vi "Base File Path.vi"() -> (3 "Paths Out":T1)   [LabVIEW 2018]
uses:
  File Paths.ctl
panel:
  in  "Paths":T1
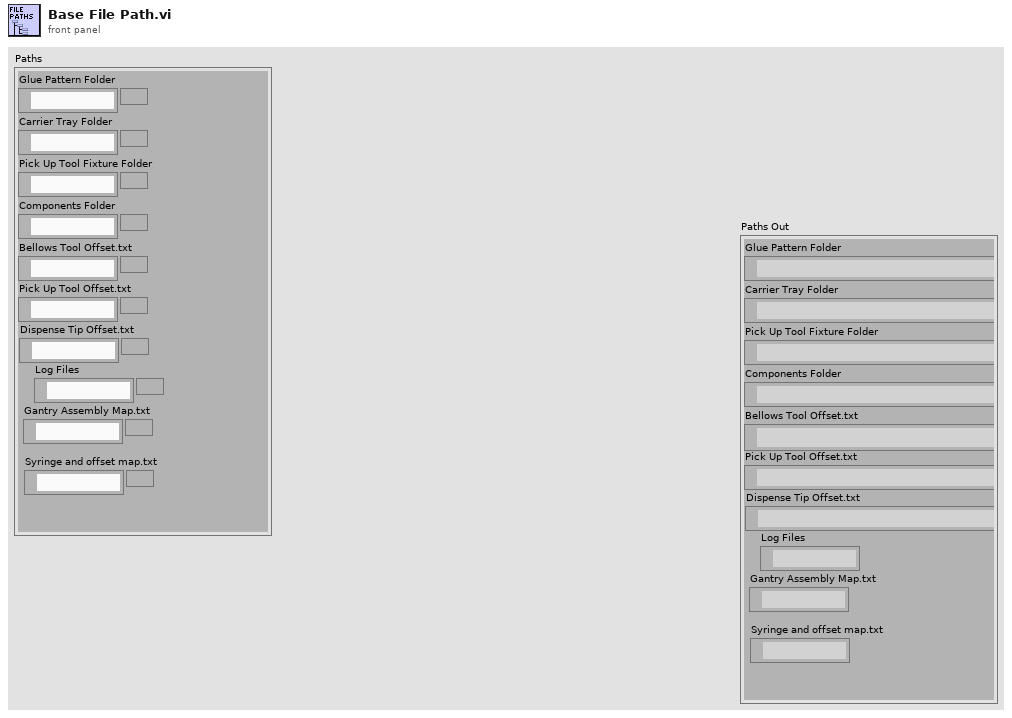
[diagram p1: front panel]
types:
  T1 = typedef "File Paths.ctl" = cluster{"Glue Pattern Folder":path, "Carrier Tray Folder":path, "Pick Up Tool Fixture Folder":path, "Components Folder":path, "Bellows Tool Offset.txt":path, "Pick Up Tool Offset.txt":path, "Dispense Tip Offset.txt":path, "Log Files":path, "Gantry Assembly Map.txt":path, "Syringe and offset map.txt":path}
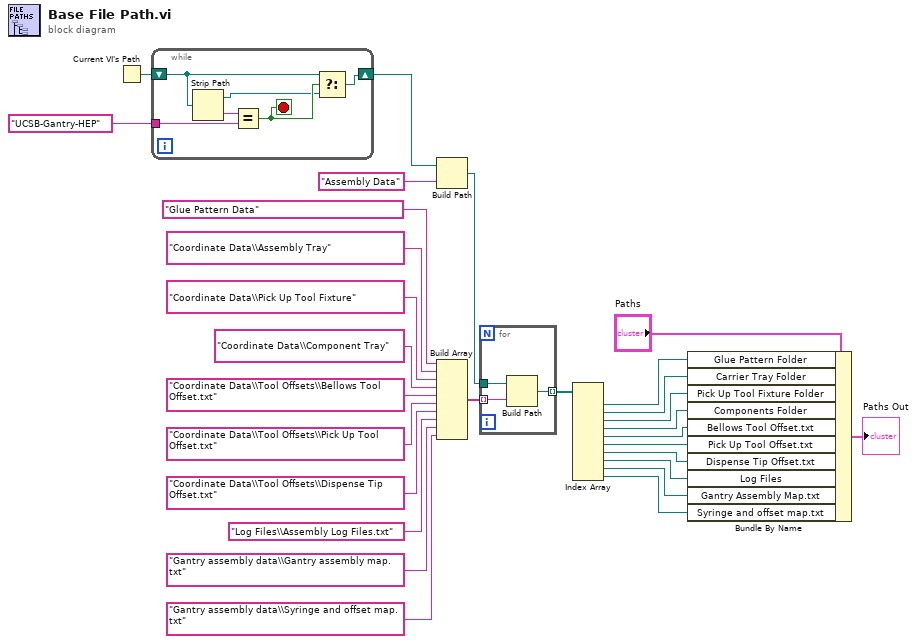
[diagram p0: block diagram]
diagram:
  n1 = Current VI's Path() -> (path=w29:path)
  n2 = while {
    shift-right: [w31] -> w25
    shift-left: w29 -> [w33]
    tunnel: "UCSB-Gantry-HEP" -> [w30]
    stop <- w34 stop-if-true
    n3 = Strip Path(path=w33) -> (stripped path=w32:path, name=w35:string)
    n4 = Equal?(x=w35, y=w30) -> (x = y?=w34:bool)
    n5 = Select(t=w33, s=w34, f=w32) -> (s? t:f=w31:path)
  }
  n6 = Build Path(base path=w25, name or relative path="Assembly Data") -> (appended path=w23:path)
  n7 = Build Array("Glue Pattern Data", "Coordinate Data\\Assembly Tray", "Coordinate Data\\Pick Up Tool Fixture", "Coordinate Data\\Component Tray" ("element"), "Coordinate Data\\Tool Offsets\\Bellows Tool Offset.txt", "Coordinate Data\\Tool Offsets\\Pick Up Tool Offset.txt", "Coordinate Data\\Tool Offsets\\Dispense Tip Offset.txt", "Log Files\\Assembly Log Files.txt", "Gantry assembly data\\Gantry assembly map.txt", "Gantry assembly data\\Syringe and offset map.txt") -> (w15:string[])
  n8 = for {
    tunnel: w23 -> [w38]
    tunnel: [w37] -> w27 mode=indexing
    tunnel: w15 -> [w36] mode=indexing
    n9 = Build Path(base path=w38, name or relative path=w36) -> (appended path=w37:path)
  }
  n10 = Index Array(array=w27) -> (element #1=w14:path, element #2=w13:path, element #3=w12:path, element #4=w11:path, element #5=w10:path, element #6=w9:path, element #7=w8:path, element #8=w5:path, element #9=w2:path, element #10=w1:path)  [unwired: 10 in]
  n11 = Bundle By Name(cluster="Paths", "Glue Pattern Folder"=w14, "Carrier Tray Folder"=w13, "Pick Up Tool Fixture Folder"=w12, "Components Folder"=w11, "Bellows Tool Offset.txt"=w10, "Pick Up Tool Offset.txt"=w9, "Dispense Tip Offset.txt"=w8, "Log Files"=w5, "Gantry Assembly Map.txt"=w2, "Syringe and offset map.txt"=w1) -> (→"Paths Out":T1)
